vi "CTRE_Phoenix_PigeonIMU_GetStatusFramePeriod.vi"(6 "timeoutMs":u32, 8 "error in":errorcluster, 10 "Pigeon IMU Status Frame":T1=270336 items=["CondStatus_1_General"=270336, "CondStatus_9_SixDeg_YPR"=270848, "CondStatus_6_SensorFusion"=270656, "CondStatus_11_GyroAccum"=270976, "CondStatus_2_GeneralCompass"=270400, "CondStatus_3_GeneralAccel"=270464, "CondStatus_10_SixDeg_Quat"=270912, "RawStatus_4_Mag"=265408, "BiasedStatus_2_Gyro"=269376, "BiasedStatus_4_Mag"=269504, "BiasedStatus_6_Accel"=269632], 11 "CTRE_PigeonIMU_DeviceRef":T2={"DeviceStatus"={"status"=FALSE, "code"=0, "source"=""}, "Device Number"=0, "Type"=352321536, "Device ID"=0, "Handle"=0, "UsageFrame"=0, "Library Path"=path ""} {"Type" items=["CAN"=352321536, "TalonSRX"=33554432]}) -> (0 "error out":errorcluster, 2 "periodMs":u32, 3 "CTRE_PigeonIMU_DeviceRef":T2={"DeviceStatus"={"status"=FALSE, "code"=0, "source"=""}, "Device Number"=0, "Type"=352321536, "Device ID"=0, "Handle"=0, "UsageFrame"=0, "Library Path"=path ""} {"Type" items=["CAN"=352321536, "TalonSRX"=33554432]})   [LabVIEW 2017]
doc: "Returns the period of the selected Status Frame."
uses:
  CTRE_PigeonIMU_DeviceRef.ctl
  CTRE_PigeonIMU_ConnectionType.ctl
  CTRE_PigeonIMU_StatusFrameRate.ctl
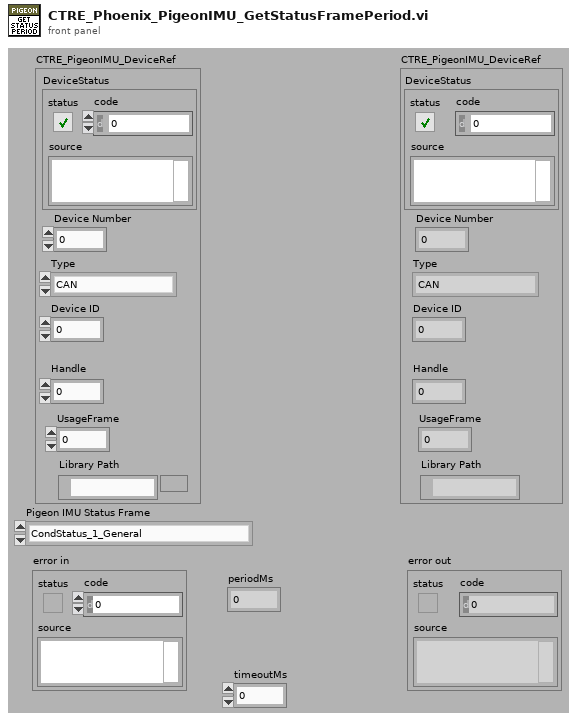
[diagram p1: front panel]
types:
  T1 = typedef "CTRE_PigeonIMU_StatusFrameRate.ctl" = u32
  T2 = typedef "CTRE_PigeonIMU_DeviceRef.ctl" = cluster{"DeviceStatus":errorcluster, "Device Number":u8, "Type":T3, "Device ID":u32, "Handle":u64, "UsageFrame":u32, "Library Path":path}
  T3 = typedef "CTRE_PigeonIMU_ConnectionType.ctl" = u32
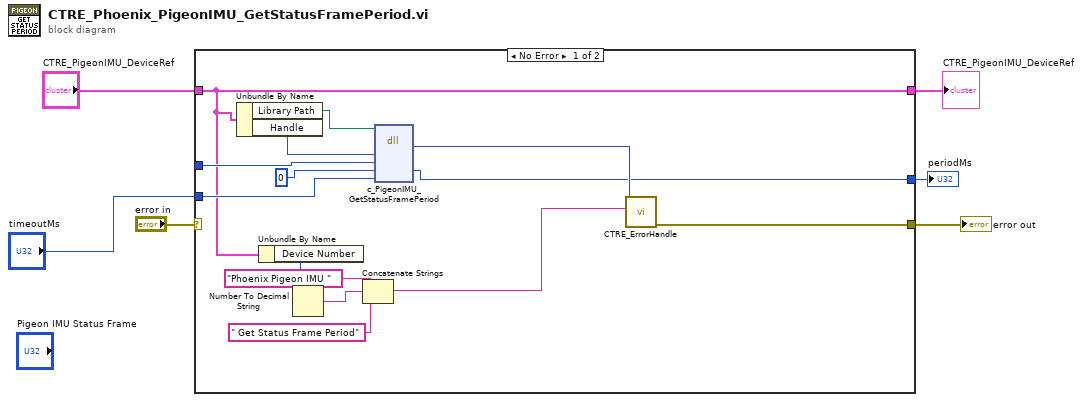
[diagram p0: block diagram]
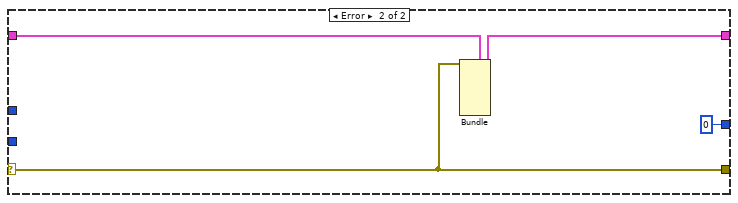
[diagram p2: hidden frame]
diagram:
  n1 = case shown="No Error" "error in" {
    selector: "error in" -> [_ w24]
    tunnel: "CTRE_PigeonIMU_DeviceRef" -> [w10 w25]
    tunnel: [w20 w24] -> w7
    tunnel: [w10 w23] -> w2
    tunnel: [w13 0 ("percentOutput")] -> w5
    tunnel: "timeoutMs" -> [w12 _]
    tunnel: [w11 _] -> w1
    frame No Error {
      n2 = Unbundle By Name(w10) -> ("Library Path"=w9:path, "Handle"=w8:u64)
      n3 = Unbundle By Name(w10) -> ("Device Number"=w16:u8)
      n4 = Number To Decimal String(number=w16) -> (decimal integer string=w18:string)  [unwired: 1 in]
      n5 = Concatenate Strings("Phoenix Pigeon IMU " ("string"), w18, " Get Status Frame Period" ("string")) -> (w14:string)
      n6 = dll-call lib="?" fn="c_PigeonIMU_GetStatusFramePeriod"(path in=w9, "handle"=w8, "frame"=w11, "periodMs"=u32 0 ("appliedThrottle"), "timeoutMs"=w12) -> ("return type"=w15:i32, "periodMs"=w13:u32)  [unwired: 5 in, 2 out]
      n7 = call "CTRE_ErrorHandle.vi"("origin"=w14, "code"=w15) -> ("error out"=w20:errorcluster)  [unwired: 9 in]
    }
    frame Error {
      n8 = Bundle(cluster=w25, "DeviceStatus"=w24) -> (w23:T2)  [unwired: 6 in]
    }
  }
  "error out" <- w7
  "periodMs" <- w5
  "CTRE_PigeonIMU_DeviceRef" <- w2
